vi "Read Waveform.vi"(8 "Error In":errorcluster, 11 "reference in":refnum<class "Scope Base.lvclass">) -> (0 "Error Out":errorcluster, 2 "Waveform":waveform(dbl), 3 "reference out":refnum<class "Scope Base.lvclass">)   [LabVIEW 2023, in "Scope Base.lvlib" / "Scope Base.lvclass"]
uses:
  Scope Base.lvclass
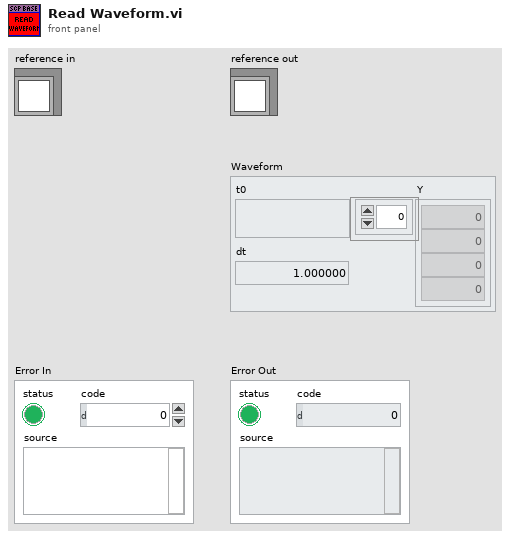
[diagram p1: front panel]
types:
  T1 = typedef "Scope Base.lvlib/Scope Base.lvclass/ObjectAttributes.ctl" = cluster{"Last Waveforms":map{u8, waveform(dbl)}}
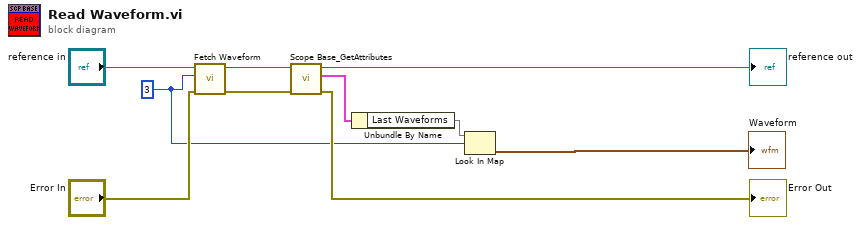
[diagram p0: block diagram]
diagram:
  w3 = u8 3 ("Channel")
  n1 = call-dynamic "Fetch Waveform.vi"("Error In"="Error In", "Channel"=w3, "reference in"="reference in") -> ("Error Out"=w5:errorcluster, "reference out"=w4:refnum<class "Scope Base.lvclass">)  [unwired: 7 in]
  n2 = call "Scope Base_GetAttributes.vi"("Error In"=w5, "reference in"=w4) -> ("Error Out"=→"Error Out":errorcluster, "Data"=w1:T1, "reference out"=→"reference out":refnum<class "Scope Base.lvclass">)  [unwired: 6 in, 1 out]
  n3 = Unbundle By Name(w1) -> ("Last Waveforms"=w2:map{u8, waveform(dbl)})
  n4 = Look In Map(map=w2, key=w3) -> (value=→"Waveform":waveform(dbl))  [unwired: 1 in, 1 out]
